vi "Save JUnit Report.vi"(8 "Error In (No Error)":errorcluster, 10 "XML file path":path, 11 "File Ref In":refnum<k20>) -> (0 "Error Out":errorcluster)   [LabVIEW 2013, in "JUnit API.lvlib"]
uses:
  JUnit API.lvlib
  <vilib>/xml/Close Reference(Node).vi
  <vilib>/xml/NI_XML.lvlib
  <vilib>/NI/Simple XML/Simple XML.lvlib
  <resource>/objmgr/DOMUserDefRef.rc
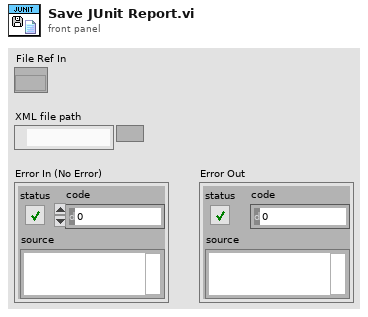
[diagram p1: front panel]
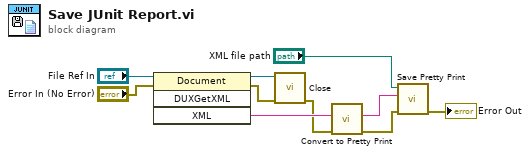
[diagram p0: block diagram]
diagram:
  n1 = invoke class="Document" method="DUXGetXML"(reference="File Ref In", error in="Error In (No Error)") -> (reference out=w6:refnum<k20>, error out=w9:errorcluster, "XML"=w2:string)  [unwired: 2 in, 1 out]
  n2 = call-poly <vilib>:"Close.vi"("error in (no error)"=w9, "node"=w6) -> ("error out"=w1:errorcluster)  [unwired: 7 in]
  n3 = call <vilib>:"Convert to Pretty Print.vi"("error in (no error)"=w1, "XML String"=w2) -> ("error out"=w5:errorcluster, "Pretty XML String"=w4:string)  [unwired: 8 in]
  n4 = call <vilib>:"Save Pretty Print.vi"("error in (no error)"=w5, "Pretty XML String"=w4, "XML file path"="XML file path") -> ("error out"=→"Error Out":errorcluster)  [unwired: 7 in, 1 out]
